vi "getPDFData.vi"(0 "reference in":refnum<class "checkIN.lvclass">, 1 "file (use dialog)":path, 5 "error in (no error)":errorcluster) -> (14 "reference out":refnum<class "checkIN.lvclass">, 16 "dataOUT":T1, 19 "error out":errorcluster)   [LabVIEW 2014, in "checkIN.lvclass"]
uses:
  checkIN.lvclass
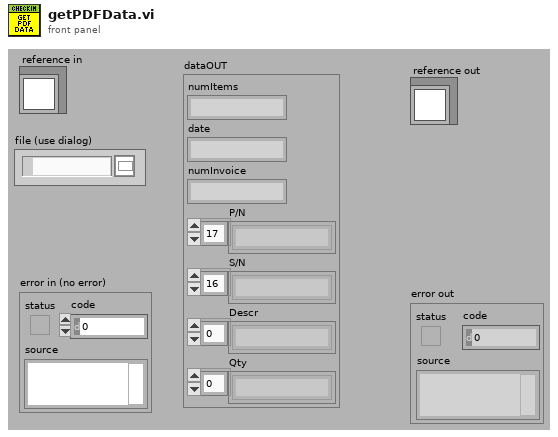
[diagram p1: front panel]
types:
  T1 = cluster{"numItems":string, "date":string, "numInvoice":string, "P/N":string[], "S/N":string[], "Descr":string[], "Qty":string[]}
  T2 = enum16{"date", "numItems", "numInvoice", "DataWithQty", "DataNoQty", "NextData", "Stop"}
  T3 = typedef "checkIN.lvclass/ObjectAttributesRef.ctl" = refnum<data-value>
  T4 = typedef "checkIN.lvclass/ObjectAttributes.ctl" = cluster{"MyAttribute":dbl, "data":string[][], "checkIN.lvclass":refnum<class "checkIN.lvclass">}
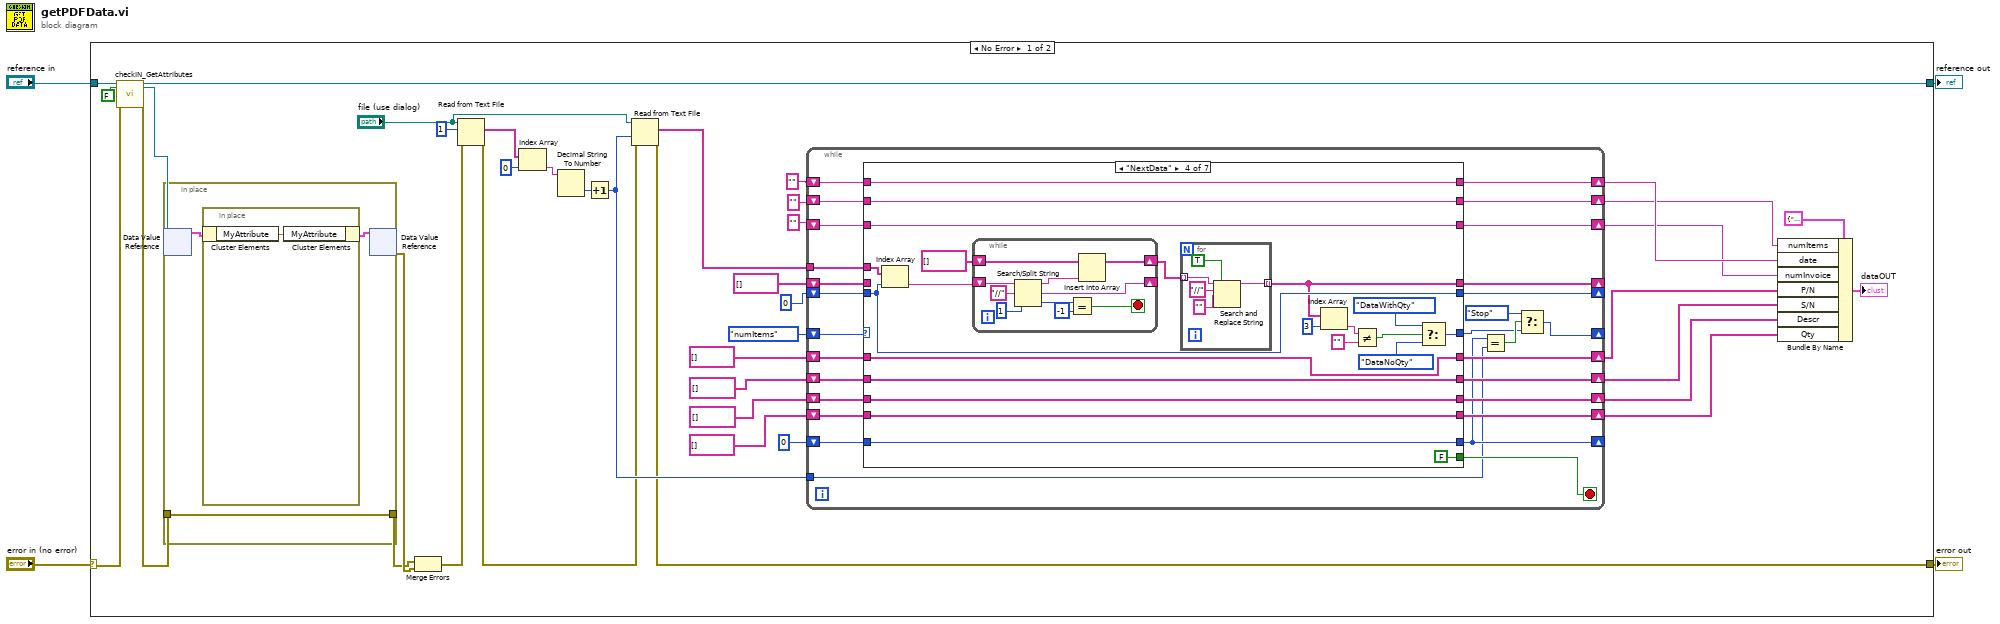
[diagram p0: block diagram]
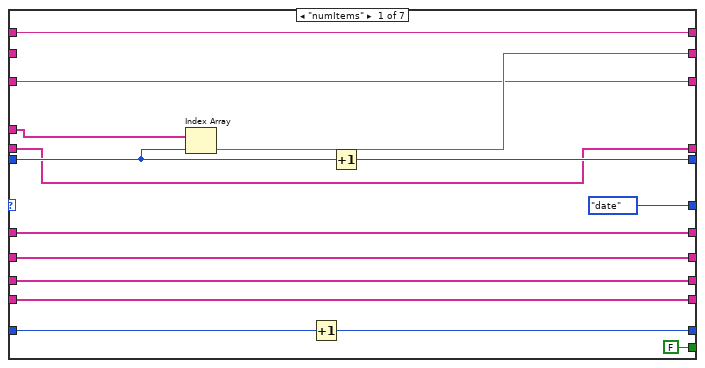
[diagram p2: hidden frame]
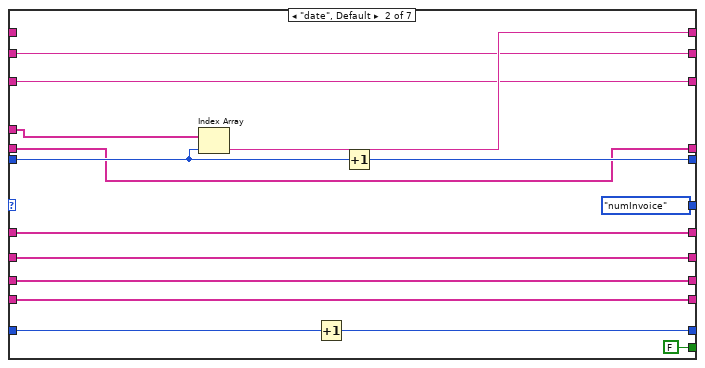
[diagram p3: hidden frame]
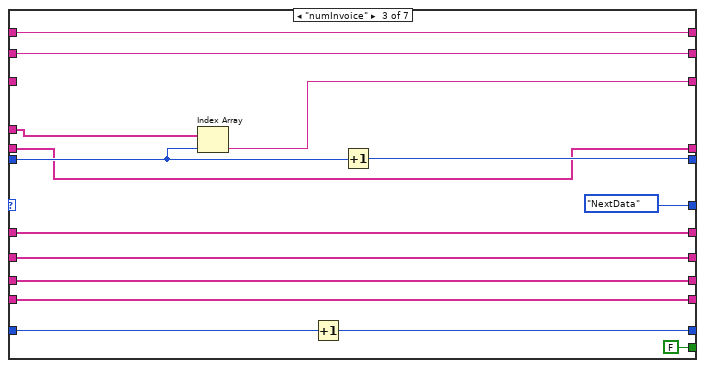
[diagram p4: hidden frame]
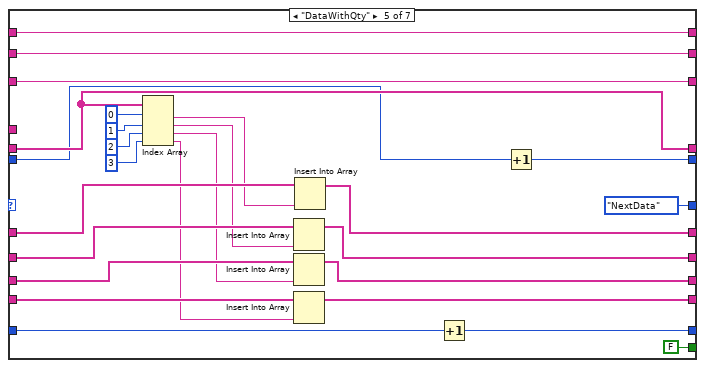
[diagram p5: hidden frame]
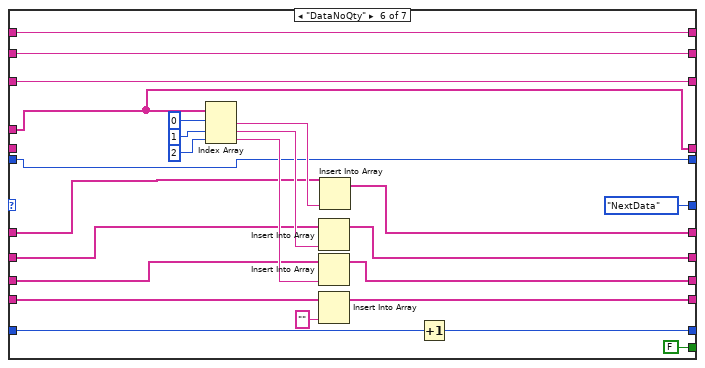
[diagram p6: hidden frame]
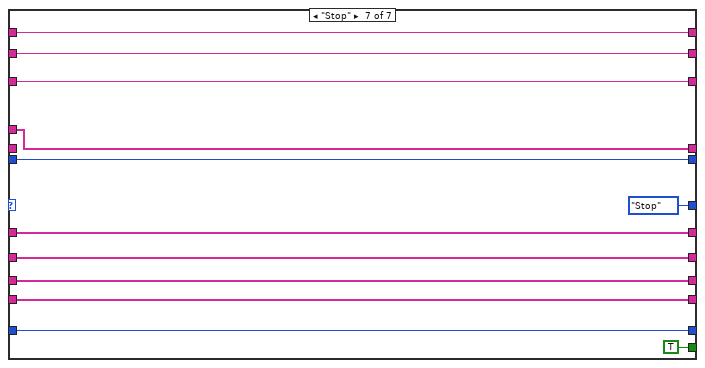
[diagram p7: hidden frame]
diagram:
  n1 = case shown="No Error" "error in (no error)" {
    selector: "error in (no error)" -> [w39 w221]
    tunnel: [w15 w221] -> w3
    tunnel: [w37 w220] -> w1
    tunnel: "reference in" -> [w41 w220]
    frame No Error {
      n2 = call "checkIN_GetAttributes.vi"("reference in"=w41, "return data? (T)"=FALSE, "error in (no error)"=w39) -> ("reference out"=w37:refnum<class "checkIN.lvclass">, "attributes ref"=w36:T3, "error out"=w38:errorcluster)  [unwired: 13 in, 1 out]
      n3 = in-place {
        in-place-border: w38 -> [w216]
        in-place-border: [w216] -> w42
        n4 = in-place-dvr #1(w36) -> (w217:T4)  [unwired: 1 out]
        n5 = in-place {
          n6 = in-place-cluster #2(w217) -> ("MyAttribute"=w219:dbl)
          n7 = in-place-cluster #2("MyAttribute"=w219) -> (w218:T4)
        }
        n8 = in-place-dvr #1(w218) -> (w43:errorcluster)  [unwired: 1 out]
      }
      n9 = Merge Errors(w42, w43) -> (w22:errorcluster)
      n10 = Read from Text File(file (use dialog)="file (use dialog)", count=1, error in=w22) -> (text=w21:string[], error out=w16:errorcluster)  [unwired: 1 in, 2 out]
      n11 = Index Array(array=w21, index=0) -> (element=w19:string)
      n12 = Decimal String To Number(string=w19) -> (number=w18:i32)  [unwired: 2 in, 1 out]
      n13 = Increment(x=w18) -> (x+1=w17:i32)
      n14 = Read from Text File(file (use dialog)="file (use dialog)", count=w17, error in=w16) -> (text=w35:string[], error out=w15:errorcluster)  [unwired: 1 in, 2 out]
      n15 = while {
        tunnel: w35 -> [w71]
        shift-right: [w45] -> _
        shift-left: T2."numItems" -> [w70]
        shift-right: [w67] -> _
        shift-left: 0 -> [w69]
        shift-right: [w68] -> w13
        shift-left: "" -> [w65]
        shift-right: [w66] -> w12
        shift-left: "" -> [w64]
        shift-right: [w63] -> w11
        shift-left: "" -> [w62]
        shift-right: [w61] -> _
        shift-left: string[] [] -> [w60]
        shift-right: [w49] -> _
        shift-left: 0 -> [w59]
        shift-right: [w54] -> w10
        shift-left: string[] [] -> [w58]
        shift-right: [w53] -> w9
        shift-left: string[] [] -> [w57]
        shift-right: [w52] -> w8
        shift-left: string[] [] -> [w56]
        shift-right: [w51] -> w7
        shift-left: string[] [] -> [w55]
        tunnel: w17 -> [w48]
        stop <- w50 stop-if-true
        n16 = case shown="\"NextData\"" w70 {
          tunnel: w71 -> [w86 w101 w115 w135 _ w184 w212]
          tunnel: w69 -> [w85 w95 w116 w131 w156 w183 w211]
          tunnel: [w83 w100 w114 w138 w179 w203 w215] -> w68
          tunnel: [w81 w99 w111 w131 w155 w183 w211] -> w67
          tunnel: [T2."date" T2."numInvoice" T2."NextData" w128 T2."NextData" T2."NextData" T2."Stop"] -> w46
          tunnel: [w84 w97 w113 w137 w178 w202 w214] -> w66
          tunnel: w65 -> [w83 _ w114 w138 w179 w203 w215]
          tunnel: w64 -> [_ w97 w113 w137 w178 w202 w214]
          tunnel: [w80 w96 w112 w136 w177 w201 w213] -> w63
          tunnel: w62 -> [w80 w96 _ w136 w177 w201 w213]
          tunnel: [w79 w94 w109 w130 w158 w184 w212] -> w61
          tunnel: w60 -> [w79 w94 w109 _ w158 _ _]
          tunnel: w59 -> [w78 w93 w108 w122 w176 w200 w204]
          tunnel: [w72 w87 w102 w122 w175 w180 w204] -> w49
          tunnel: w58 -> [w77 w92 w107 w121 w170 w193 w209]
          tunnel: w57 -> [w76 w91 w106 w120 w169 w192 w208]
          tunnel: w56 -> [w75 w90 w105 w119 w168 w191 w207]
          tunnel: w55 -> [w74 w89 w104 w118 w167 w190 w206]
          tunnel: [w77 w92 w107 w121 w162 w185 w209] -> w54
          tunnel: [w76 w91 w106 w120 w161 w186 w208] -> w53
          tunnel: [w75 w90 w105 w119 w160 w187 w207] -> w52
          tunnel: [w74 w89 w104 w118 w159 w188 w206] -> w51
          tunnel: [FALSE FALSE FALSE FALSE FALSE FALSE TRUE] -> w50
          frame "numItems" {
            n17 = Index Array(array=w86, index=w85) -> (element=w84:string)
            n18 = Increment(x=w78) -> (x+1=w72:i32)
            n19 = Increment(x=w85) -> (x+1=w81:i32)
          }
          frame "date", Default {
            n20 = Index Array(array=w101, index=w95) -> (element=w100:string)
            n21 = Increment(x=w93) -> (x+1=w87:i32)
            n22 = Increment(x=w95) -> (x+1=w99:i32)
          }
          frame "numInvoice" {
            n23 = Index Array(array=w115, index=w116) -> (element=w112:string)
            n24 = Increment(x=w108) -> (x+1=w102:i32)
            n25 = Increment(x=w116) -> (x+1=w111:i32)
          }
          frame "NextData" {
            n26 = Index Array(array=w135, index=w131) -> (element=w133:string)
            n27 = while {
              shift-right: [w152] -> w132
              shift-left: string[] [] -> [w153]
              shift-right: [w148] -> _
              shift-left: w133 -> [w151]
              stop <- w146 stop-if-true
              n28 = Search/Split String(string=w151, search string/char (-)="//", offset (0)=1) -> (substring before match=w150:string, match + rest of string=w148:string, offset of match=w147:i32)
              n29 = Equal?(x=w147, y=-1) -> (x = y?=w146:bool)
              n30 = Insert Into Array(array=w153, new element=w150) -> (w152:string[])  [unwired: 1 in]
            }
            n31 = for {
              tunnel: [w140] -> w130 mode=indexing
              tunnel: w132 -> [w139] mode=indexing
              n32 = Search and Replace String(replace all?=TRUE ("replace all? (F)"), input string=w139, search string="//", replace string="" ("replace string (\"\")")) -> (result string=w140:string)  [unwired: 4 in, 3 out]
            }
            n33 = Index Array(array=w130, index=3) -> (element=w127:string)
            n34 = Not Equal?(x=w127, y="") -> (x != y?=w125:bool)
            n35 = Select(t=T2."DataWithQty", s=w125, f=T2."DataNoQty") -> (s? t:f=w128:T2)
          }
          frame "DataWithQty" {
            n36 = Index Array(array=w158, index #1=0, index #2=1, index #3=2, index #4=3) -> (element #1=w166:string, element #2=w165:string, element #3=w164:string, element #4=w163:string)
            n37 = Insert Into Array(array=w169, new element=w165) -> (w161:string[])  [unwired: 1 in]
            n38 = Insert Into Array(array=w168, new element=w164) -> (w160:string[])  [unwired: 1 in]
            n39 = Insert Into Array(array=w167, new element=w163) -> (w159:string[])  [unwired: 1 in]
            n40 = Insert Into Array(array=w170, new element=w166) -> (w162:string[])  [unwired: 1 in]
            n41 = Increment(x=w176) -> (x+1=w175:i32)
            n42 = Increment(x=w156) -> (x+1=w155:i32)
          }
          frame "DataNoQty" {
            n43 = Index Array(array=w184, index #1=0, index #2=1, index #3=2) -> (element #1=w196:string, element #2=w195:string, element #3=w194:string)
            n44 = Insert Into Array(array=w192, new element=w195) -> (w186:string[])  [unwired: 1 in]
            n45 = Insert Into Array(array=w191, new element=w194) -> (w187:string[])  [unwired: 1 in]
            n46 = Insert Into Array(array=w190, new element="" ("new element/subarray")) -> (w188:string[])  [unwired: 1 in]
            n47 = Insert Into Array(array=w193, new element=w196) -> (w185:string[])  [unwired: 1 in]
            n48 = Increment(x=w200) -> (x+1=w180:i32)
          }
          frame "Stop" {
          }
        }
        n49 = Equal?(x=w49, y=w48) -> (x = y?=w47:bool)
        n50 = Select(t=T2."Stop", s=w47, f=w46) -> (s? t:f=w45:T2)
      }
      n51 = Bundle By Name(cluster=T1 {"numItems"="", "date"="", "numInvoice"="", "P/N"=[], "S/N"=[], "Descr"=[], "Qty"=[]}, "numItems"=w12, "date"=w13, "numInvoice"=w11, "P/N"=w10, "S/N"=w9, "Descr"=w8, "Qty"=w7) -> (→"dataOUT":T1)
    }
    frame Error {
    }
  }
  "error out" <- w3
  "reference out" <- w1
